vi "ExternalQueue.vi"(2 "Mode":T1(ring), 5 "Queue In":string, 11 "error in (no error)":errorcluster) -> (6 "Queue Out":string, 15 "error out":errorcluster)   [LabVIEW 2011]
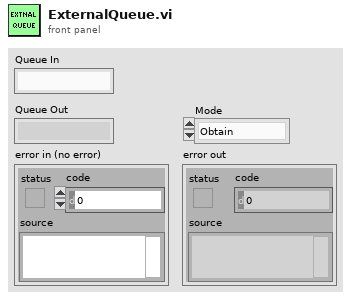
[diagram p1: front panel]
types:
  T1 = enum16{"Obtain", "Enqueue", "Dequeue", "Release"}
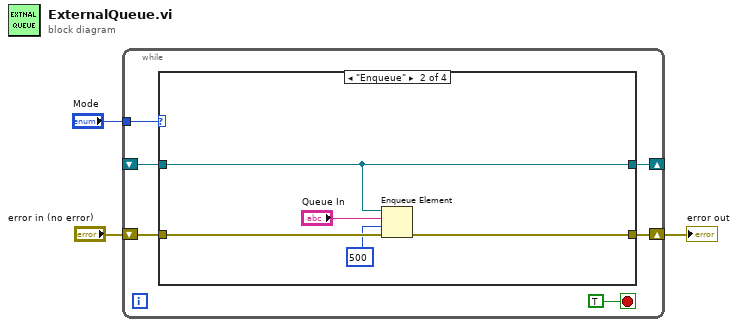
[diagram p0: block diagram]
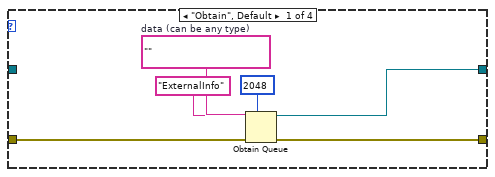
[diagram p2: hidden frame]
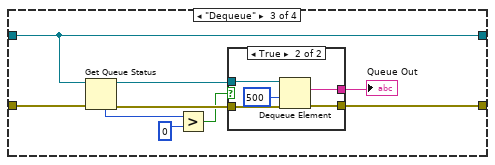
[diagram p3: hidden frame]
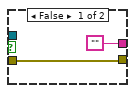
[diagram p4: hidden frame]
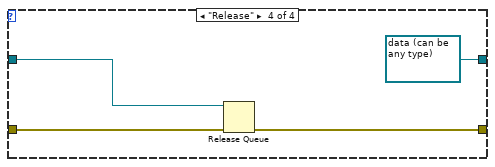
[diagram p5: hidden frame]
diagram:
  n1 = while {
    tunnel: "Mode" -> [w9]
    shift-right: [w7] -> w1
    shift-left: "error in (no error)" -> [w8]
    shift-right: [w6] -> _
    shift-left: _ -> [w5]
    stop <- TRUE stop-if-true
    n2 = case shown="\"Enqueue\"" w9 {
      tunnel: w8 -> [w15 w20 w27 w40]
      tunnel: [w14 w19 w29 w39] -> w7
      tunnel: [w11 w17 w25 refnum<queue> refnum ("queue out")] -> w6
      tunnel: w5 -> [_ w17 w25 w38]
      frame "Obtain", Default {
        w13 = ""  # data (can be any type)
        n3 = Obtain Queue(max queue size (-1, unlimited)=2048, name (unnamed)="ExternalInfo", element data type=w13, error in (no error)=w15) -> (queue out=w11:refnum<queue>, error out=w14:errorcluster)  [unwired: 1 in, 1 out]
      }
      frame "Enqueue" {
        n4 = Enqueue Element(queue=w17, element="Queue In", timeout in ms (-1)=500, error in (no error)=w20) -> (error out=w19:errorcluster)  [unwired: 2 out]
      }
      frame "Dequeue" {
        n5 = Get Queue Status(queue=w25, error in (no error)=w27) -> (queue out=w24:refnum<queue>, error out=w26:errorcluster, # elements in queue=w22:i32)  [unwired: 1 in, 5 out]
        n6 = Greater?(x=w22, y=0) -> (0:w21:bool)
        n7 = case shown="True" w21 {
          tunnel: [w30 w36] -> w29
          tunnel: ["" w35] -> w28
          tunnel: w26 -> [w30 w34]
          tunnel: w24 -> [_ w33]
          frame False {
          }
          frame True {
            n8 = Dequeue Element(queue=w33, timeout in ms (-1)=500, error in (no error)=w34) -> (element=w35:string, error out=w36:errorcluster)  [unwired: 2 out]
          }
        }
        "Queue Out" <- w28
      }
      frame "Release" {
        n9 = Release Queue(queue=w38, error in (no error)=w40) -> (error out=w39:errorcluster)  [unwired: 1 in, 2 out]
      }
    }
  }
  "error out" <- w1
